vi "Up Down Counter FGV.vi"(7 "Action Selection":T1=enum."Increment", 8 "Error In":errorcluster) -> (0 "Error Out":errorcluster, 2 "Running Total":i32)   [LabVIEW 2014]
uses:
  Up Down Counter Command.ctl
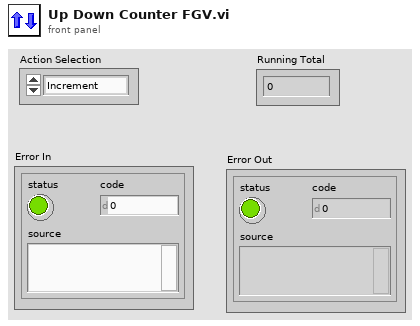
[diagram p1: front panel]
types:
  T1 = typedef "Up Down Counter Command.ctl" = enum16{"Reset", "Increment", "Decrement", "Get Current Value"}
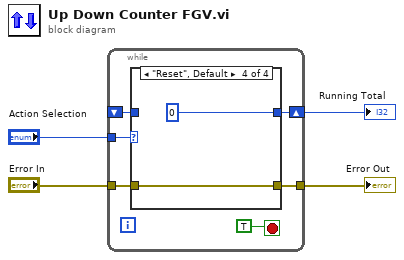
[diagram p0: block diagram]
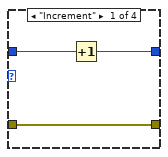
[diagram p2: hidden frame]
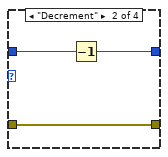
[diagram p3: hidden frame]
diagram:
  n1 = while {
    tunnel: "Action Selection" -> [w9]
    tunnel: "Error In" -> [w8]
    tunnel: [w7] -> w2
    shift-right: [w6] -> w1
    shift-left: _ -> [w5]
    stop <- TRUE stop-if-true
    n2 = case shown="\"Reset\", Default" w9 {
      tunnel: w8 -> [w13 w16 w18 w20]
      tunnel: [w13 w16 w18 w20] -> w7
      tunnel: [w11 w14 w17 0] -> w6
      tunnel: w5 -> [w12 w15 w17 _]
      frame "Increment" {
        n3 = Increment(x=w12) -> (x+1=w11:i32)
      }
      frame "Decrement" {
        n4 = Decrement(x=w15) -> (x-1=w14:i32)
      }
      frame "Get Current Value" {
      }
      frame "Reset", Default {
      }
    }
  }
  "Running Total" <- w1
  "Error Out" <- w2
